vi "AttackerAimGoalRoleVSS.vi"(8 "error in (no error)":errorcluster, 9 "Game in":refnum<class "Game.lvclass">, 11 "AttackerAimGoalRoleVSS in":refnum<class "AttackerAimGoalRoleVSS.lvclass">) -> (0 "error out":errorcluster, 1 "Game out":refnum<class "Game.lvclass">, 2 "Robot out":refnum<class "Robot.lvclass">, 3 "AttackerAimGoalRoleVSS out":refnum<class "AttackerAimGoalRoleVSS.lvclass">)   [LabVIEW 2023, in "AttackerAimGoalRoleVSS.lvclass"]
uses:
  AttackerAimGoalRoleVSS.lvclass
  Robot_class/Robot.lvclass
  Game_class/Game.lvclass
  Role_class/Role.lvclass/Role.ctl
  Role_class/Read Tacticbook.vi
  Role_class/Read tactic_index.vi
  Role_class/Write Tacticbook.vi
  Role_class/Write tactic_index.vi
  Role_class/Read RobotRef.vi
  Tacticbook_class/Tacticbook.lvclass
  DispBallTacticVSS_class/DispBallTacticVSS.lvclass
  DefendGoalTacticVSS_class/DefendGoalTacticVSS.lvclass
  PenaltyAttackTacticVSS_class/PenaltyAttackTacticVSS.lvclass
  DefendAreaTacticVSS_class/DefendAreaTacticVSS.lvclass
  AttackTacticVSS_class/AttackTacticVSS.lvclass
  HaltTactic_class/HaltTactic.lvclass
  GoAndKickTacticVSS_class/GoAndKickTacticVSS.lvclass
  GoalKickKeeperTacticVSS_class/GoalKickKeeperTacticVSS.lvclass
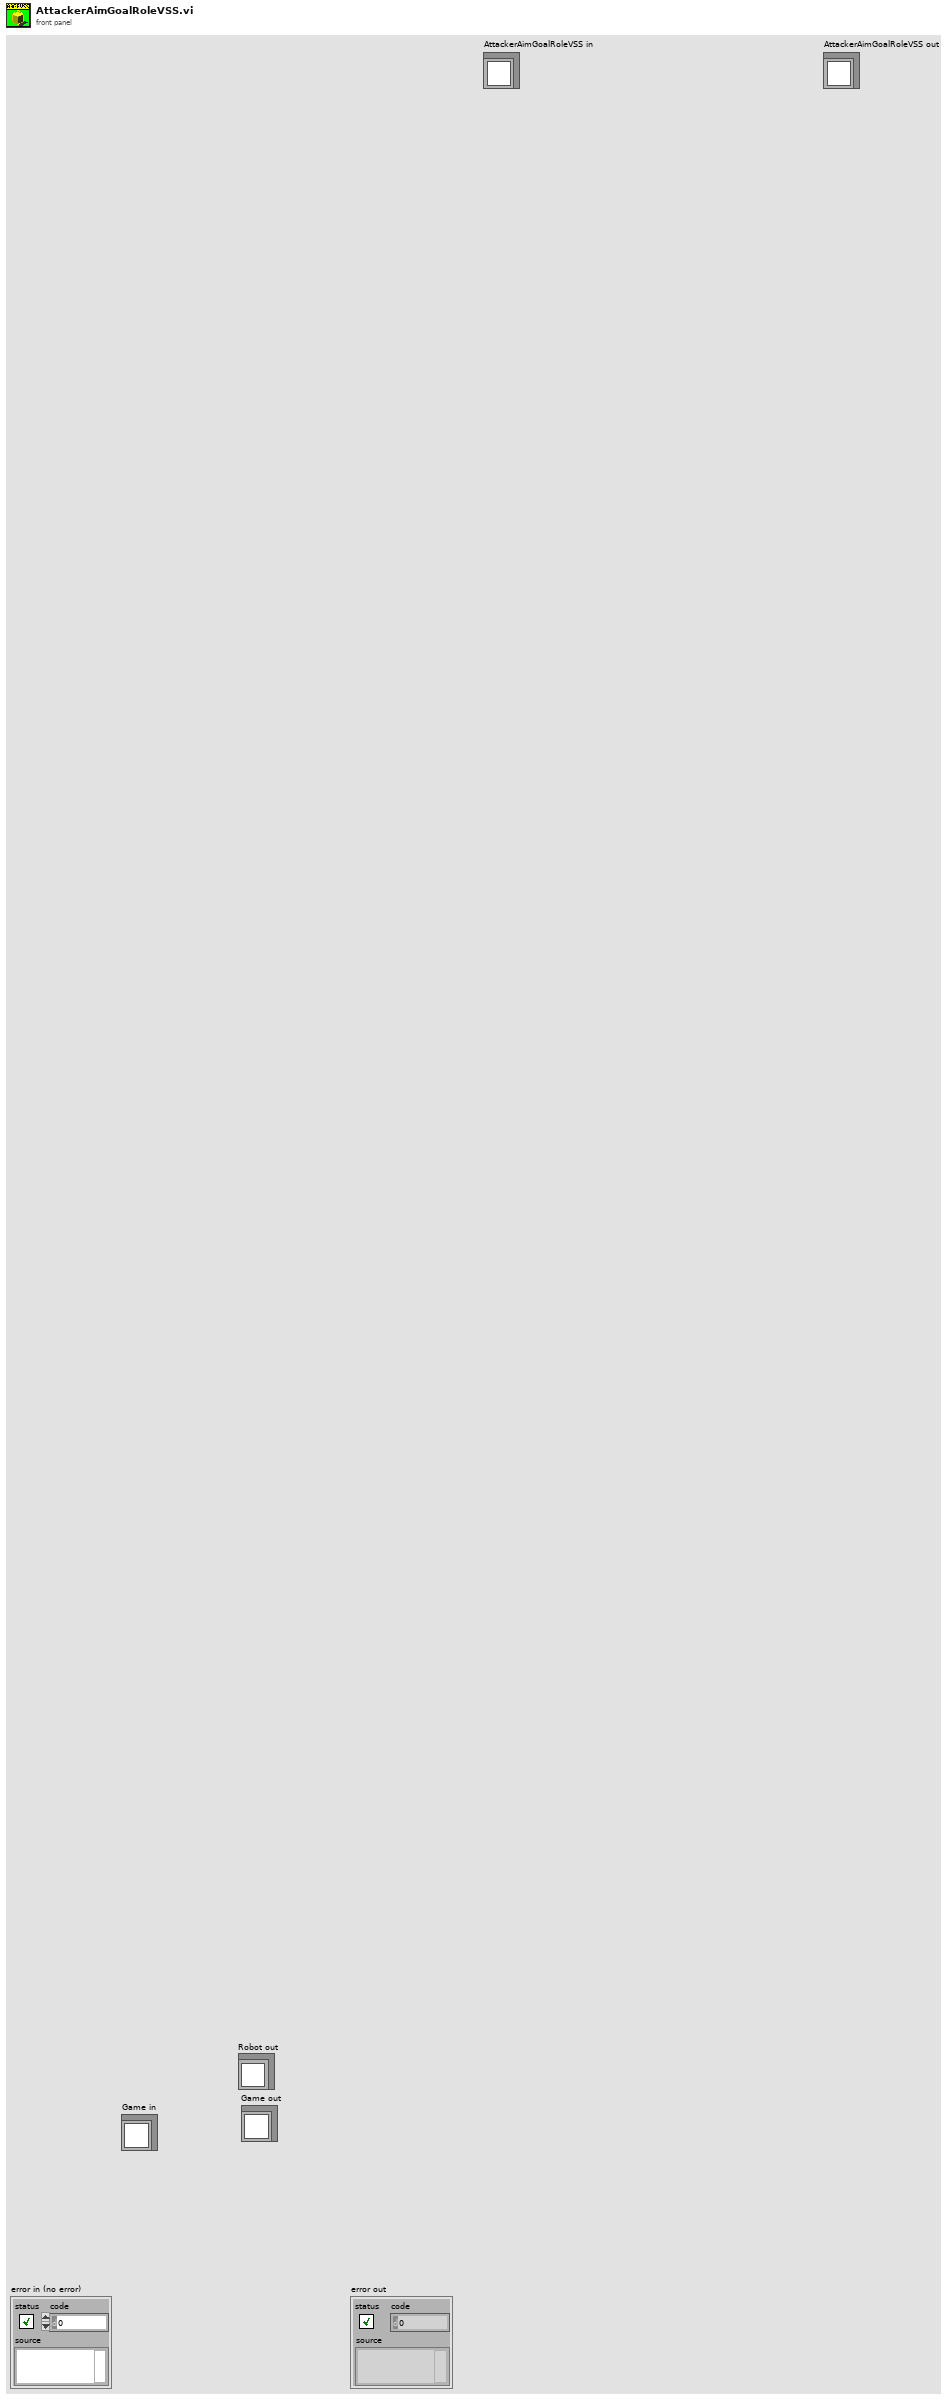
[diagram p1: front panel]
types:
  T1 = cluster{"DispBallTacticVSS":refnum<class "DispBallTacticVSS.lvclass">, "DefendGoalTacticVSS":refnum<class "DefendGoalTacticVSS.lvclass">, "PenaltyAttackTacticVSS":refnum<class "PenaltyAttackTacticVSS.lvclass">, "DefendAreaTacticVSS":refnum<class "DefendAreaTacticVSS.lvclass">, "AttackTacticVSS":refnum<class "AttackTacticVSS.lvclass">, "HaltTactic":refnum<class "HaltTactic.lvclass">, "GoAndKickTacticVSS":refnum<class "GoAndKickTacticVSS.lvclass">, "GoalKickKeeperTacticVSS":refnum<class "GoalKickKeeperTacticVSS.lvclass">}
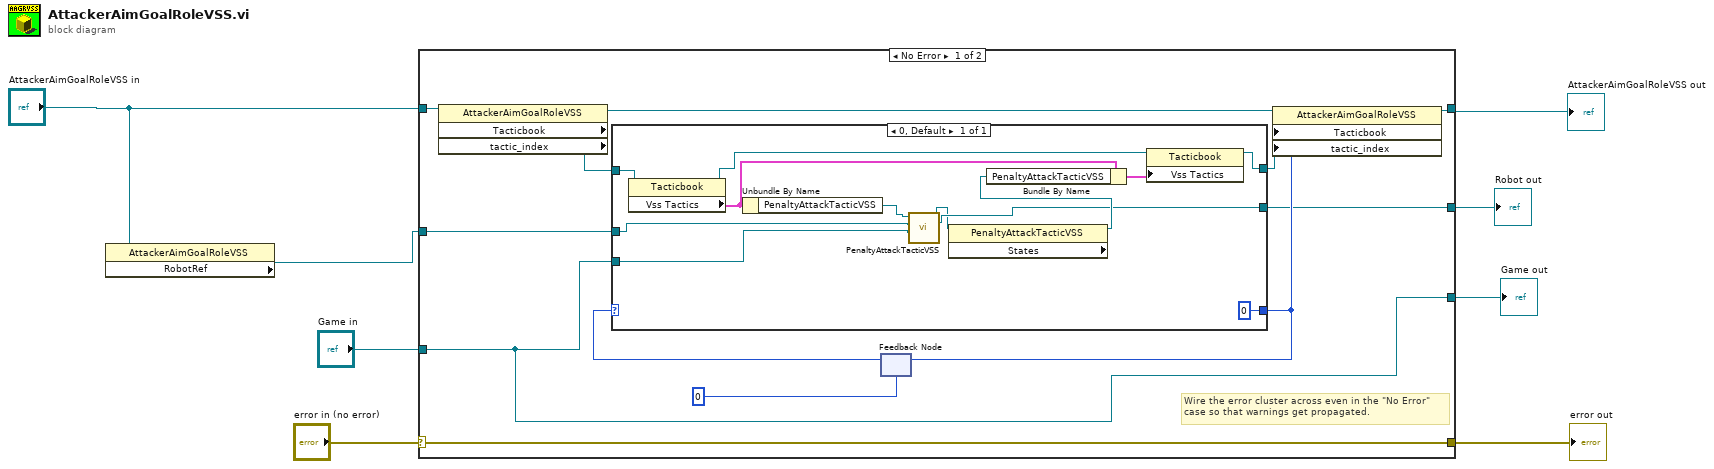
[diagram p0: block diagram]
diagram:
  n1 = property class="AttackerAimGoalRoleVSS"(reference="AttackerAimGoalRoleVSS in") -> ("RobotRef"=w3:refnum<class "Robot.lvclass">)  [unwired: 1 in, 2 out]
  n2 = case shown="No Error" "error in (no error)" {
    selector: "error in (no error)" -> [w20 w36]
    tunnel: [w20 w36] -> w7
    tunnel: [w18 w35] -> w1
    tunnel: "AttackerAimGoalRoleVSS in" -> [w19 w35]
    tunnel: w3 -> [w12 w34]
    tunnel: [w11 w34] -> w6
    tunnel: [w9 w33] -> w5
    tunnel: "Game in" -> [w9 w33]
    frame No Error {
      # "Wire the error cluster across even in the \"No Error\"\ncase so that warnings get propagated."
      n3 = property class="AttackerAimGoalRoleVSS" props=["Tacticbook", "tactic_index"](reference=w19) -> (reference out=w17:refnum<class "AttackerAimGoalRoleVSS.lvclass">, "Tacticbook"=w14:refnum<class "Tacticbook.lvclass">)  [unwired: 1 in, 2 out]
      n4 = feedback #1(0) -> (w15:i32)
      n5 = case shown="0, Default" w15 {
        tunnel: [0] -> w13
        tunnel: w14 -> [w32]
        tunnel: w12 -> [w22]
        tunnel: [w25] -> w11
        tunnel: [w30] -> w10
        tunnel: w9 -> [w21]
        frame 0, Default {
          n6 = property class="Tacticbook"(reference=w32) -> (reference out=w31:refnum<class "Tacticbook.lvclass">, "Vss Tactics"=w28:T1)  [unwired: 1 in, 1 out]
          n7 = Unbundle By Name(w28) -> ("PenaltyAttackTacticVSS"=w23:refnum<class "PenaltyAttackTacticVSS.lvclass">)
          n8 = call "PenaltyAttackTacticVSS.vi"("Game in"=w21, "Robot"=w22, "PenaltyAttackTacticVSS in"=w23) -> ("Robot out"=w25:refnum<class "Robot.lvclass">, "PenaltyAttackTacticVSS out"=w24:refnum<class "PenaltyAttackTacticVSS.lvclass">)  [unwired: 7 in]
          n9 = property class="PenaltyAttackTacticVSS" props=["States"](reference=w24) -> (reference out=w26:refnum<class "PenaltyAttackTacticVSS.lvclass">)  [unwired: 1 in, 2 out]
          n10 = Bundle By Name(cluster=w28, "PenaltyAttackTacticVSS"=w26) -> (w27:T1)
          n11 = property class="Tacticbook"(reference=w31, "Vss Tactics"=w27) -> (reference out=w30:refnum<class "Tacticbook.lvclass">)  [unwired: 1 in, 1 out]
        }
      }
      n12 = feedback-in #1(w13) -> ()
      n13 = property class="AttackerAimGoalRoleVSS"(reference=w17, "Tacticbook"=w10, "tactic_index"=w13) -> (reference out=w18:refnum<class "AttackerAimGoalRoleVSS.lvclass">)  [unwired: 1 in, 1 out]
    }
    frame Error {
    }
  }
  "AttackerAimGoalRoleVSS out" <- w1
  "error out" <- w7
  "Robot out" <- w6
  "Game out" <- w5
